vi "Close Waveform Streaming Manager Reference.vi"(8 "error in (no error)":errorcluster, 11 "WaveformStreaming":T1) -> (0 "error out":errorcluster)   [LabVIEW 2020, in "NI_VS Waveform Streaming Interface.lvlib"]
doc: "Closes an open reference to the waveform-stream manager on the VeriStand Gateway. Use this VI to close waveform-stream manager references you open with the Open Waveform Stream Manager Reference VI."
uses:
  <vilib>/NI VeriStand/Execution/WaveformStreaming/NI_VS Waveform Streaming Interface.lvlib
  <vilib>/NI VeriStand/Execution/WaveformStreaming/WaveformStreamingAPI.ctl
  NationalInstruments.VeriStand.ClientAPI
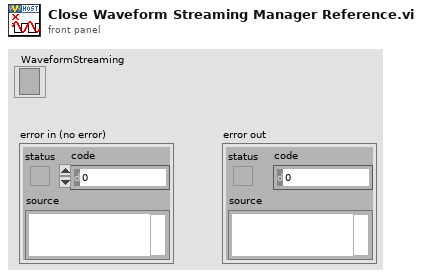
[diagram p1: front panel]
types:
  T1 = typedef "NI_VS Waveform Streaming Interface.lvlib/WaveformStreamingAPI.ctl" = refnum<k24>
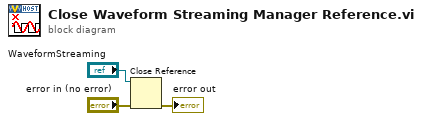
[diagram p0: block diagram]
diagram:
  n1 = Close Reference(reference="WaveformStreaming", error in (no error)="error in (no error)") -> (error out=→"error out":errorcluster)
